vi "MB Embedded Modbus Demo Box Example.vi"() -> ()   [LabVIEW 2019, in "NI_modbus_upd.lvlib"]
uses:
  NI_modbus_upd.lvlib
  Ctl/MB Modbus Command.ctl
panel:
  in  "Stop":bool
  in  "COM Port":refnum<visa-resource-name>
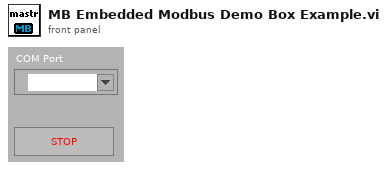
[diagram p1: front panel]
types:
  T1 = cluster{"Mode":enum16{"RTU", "ASCII"}, "Slave Address":u8}
  T2 = typedef "NI_modbus_upd.lvlib/MB Modbus Command.ctl" = cluster{"Function Code":u8, "Starting Address":u16, "Quantity":u16, "Data":u16[], "Discrete":bool[]}
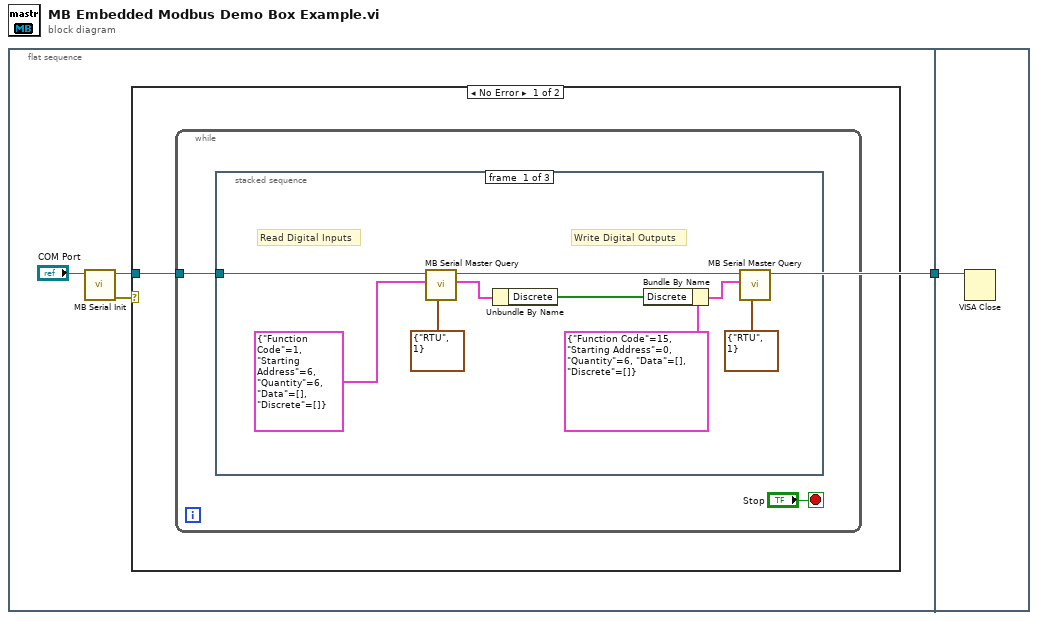
[diagram p0: block diagram]
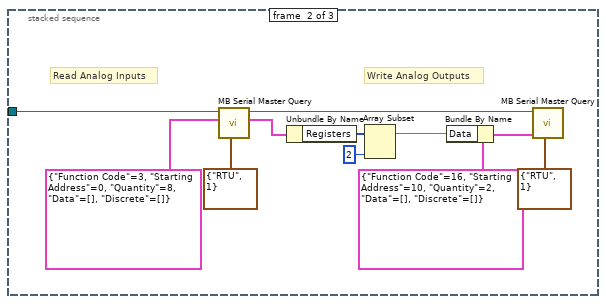
[diagram p2: hidden frame]
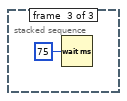
[diagram p3: hidden frame]
diagram:
  n1 = flat-sequence {
    tunnel: [w3] -> w1
    tunnel: w1 -> [w29]
    frame #0 {
      n2 = call "MB Serial Init.vi"("VISA resource name"="COM Port") -> ("error out"=w2:errorcluster, "VISA resource name out"=w3:refnum<visa-resource-name>)  [unwired: 9 in]
      n3 = case shown="No Error" w2 {
        tunnel: w3 -> [w5 _]
        frame No Error {
          n4 = while {
            tunnel: w5 -> [w7]
            stop <- "Stop" stop-if-true
            n5 = stacked-sequence {
              tunnel: w7 -> [w13 w24 _]
              frame #0 {
                # "Write Digital Outputs"
                # "Read Digital Inputs"
                n6 = call "MB Serial Master Query.vi"("Serial Parameters"=T1 {"Mode"=enum."RTU", "Slave Address"=1}, "Modbus Command"=T2 {"Function Code"=1, "Starting Address"=6, "Quantity"=6, "Data"=[], "Discrete"=[]} ("MODBUS Command"), "VISA resource name"=w13) -> ("Registers"=w16:cluster{"Registers":u16[], "Discrete":bool[]}, "VISA resource name out"=w9:refnum<visa-resource-name>)  [unwired: 4 in, 3 out]
                n7 = Unbundle By Name(w16) -> ("Discrete"=w8:bool[])
                n8 = Bundle By Name(cluster=T2 {"Function Code"=15, "Starting Address"=0, "Quantity"=6, "Data"=[], "Discrete"=[]} ("MODBUS Command"), "Discrete"=w8) -> (w10:T2)
                n9 = call "MB Serial Master Query.vi"("Serial Parameters"=T1 {"Mode"=enum."RTU", "Slave Address"=1}, "Modbus Command"=w10, "VISA resource name"=w9) -> ()  [unwired: 4 in, 5 out]
              }
              frame #1 {
                # "Write Analog Outputs"
                # "Read Analog Inputs"
                n10 = call "MB Serial Master Query.vi"("Serial Parameters"=T1 {"Mode"=enum."RTU", "Slave Address"=1}, "Modbus Command"=T2 {"Function Code"=3, "Starting Address"=0, "Quantity"=8, "Data"=[], "Discrete"=[]} ("MODBUS Command"), "VISA resource name"=w24) -> ("Registers"=w27:cluster{"Registers":u16[], "Discrete":bool[]}, "VISA resource name out"=w20:refnum<visa-resource-name>)  [unwired: 4 in, 3 out]
                n11 = Unbundle By Name(w27) -> ("Registers"=w19:u16[])
                n12 = Array Subset(array=w19, length=2) -> (w17:u16[])  [unwired: 1 in]
                n13 = Bundle By Name(cluster=T2 {"Function Code"=16, "Starting Address"=10, "Quantity"=2, "Data"=[], "Discrete"=[]} ("MODBUS Command"), "Data"=w17) -> (w21:T2)
                n14 = call "MB Serial Master Query.vi"("Serial Parameters"=T1 {"Mode"=enum."RTU", "Slave Address"=1}, "Modbus Command"=w21, "VISA resource name"=w20) -> ()  [unwired: 4 in, 5 out]
              }
              frame #2 {
                n15 = Wait (ms)(milliseconds to wait=u32 75) -> ()  [unwired: 1 out]
              }
            }
          }
        }
        frame Error {
        }
      }
    }
    frame #1 {
      n16 = VISA Close(VISA resource name=w29) -> ()  [unwired: 1 in, 1 out]
    }
  }
